vi "Start trigger export.vi"(4 "trig.pxi trig dst":i32, 6 "trig.export":T1, 7 "trig.dur":u32=25, 9 "delayed trigger":bool, 10 "synced trigger":bool, 11 "source trigger":bool) -> (0 "pxi3 ctr":u16, 1 "pxi1 ctr":u16, 2 "pxi0 ctr":u16, 3 "dst count":u16)   [LabVIEW 2019, in "FPGA Utility.lvlib"]
doc: "Handles trigger exporting to PXI tirg line"
uses:
  FPGA Utility.lvlib
  FPGA driver trigger destination.ctl
  <instrlib>/_niInstr/Basic Elements/v1/FPGA/Private/Count Up U16.vi
  <instrlib>/_niInstr/Basic Elements/v1/FPGA/niInstr Basic Elements v1 FPGA.lvlib
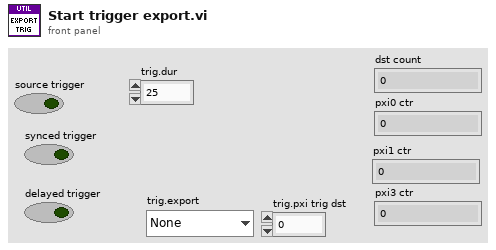
[diagram p1: front panel]
types:
  T1 = typedef "FPGA Utility.lvlib/FPGA driver trigger destination.ctl" = enum16{"None", "Source trig", "Synced trig", "Delayed sync"}
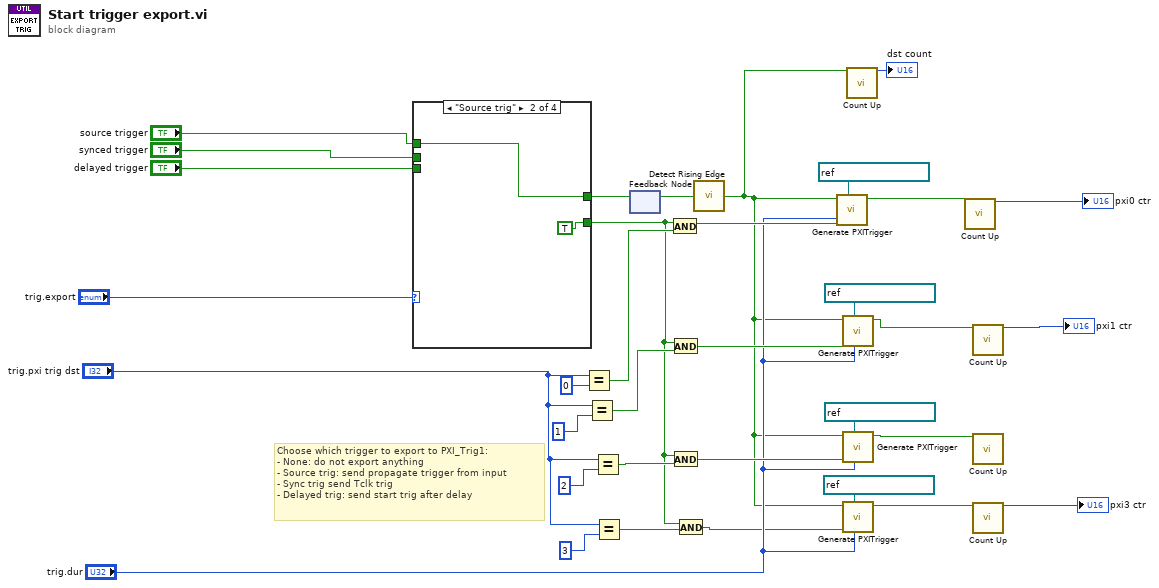
[diagram p0: block diagram]
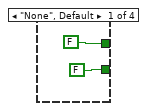
[diagram p2: hidden frame]
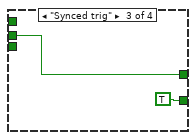
[diagram p3: hidden frame]
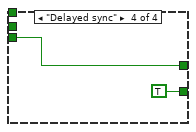
[diagram p4: hidden frame]
diagram:
  # "Choose which trigger to export to PXI_Trig1:\n- None: do not export anything\n- Source trig: send propagate trigger from input\n- Sync trig send Tclk trig\n- Delayed trig: send start trig after delay"
  n1 = case shown="\"Source trig\"" "trig.export" {
    tunnel: [FALSE TRUE TRUE TRUE] -> w6
    tunnel: [FALSE w38 w40 w41] -> w23
    tunnel: "source trigger" -> [_ w38 _ _]
    tunnel: "synced trigger" -> [_ _ w40 _]
    tunnel: "delayed trigger" -> [_ _ _ w41]
    frame "None", Default {
    }
    frame "Source trig" {
    }
    frame "Synced trig" {
    }
    frame "Delayed sync" {
    }
  }
  n2 = Equal?(x="trig.pxi trig dst", y=0) -> (x = y?=w31:bool)
  n3 = Equal?(x="trig.pxi trig dst", y=1) -> (x = y?=w33:bool)
  n4 = Equal?(x="trig.pxi trig dst", y=2) -> (x = y?=w7:bool)
  n5 = Equal?(x="trig.pxi trig dst", y=3) -> (x = y?=w5:bool)
  n6 = feedback #1() -> (w28:bool)  [unwired: 1 in]
  n7 = feedback-in #1(w23) -> ()
  n8 = And(x=w6, y=w31) -> (x .and. y?=w29:bool)
  n9 = And(x=w6, y=w33) -> (x .and. y?=w34:bool)
  n10 = And(x=w6, y=w7) -> (x .and. y?=w4:bool)
  n11 = And(x=w6, y=w5) -> (x .and. y?=w1:bool)
  n12 = call <instrlib>:"Detect Rising Edge.vi"("signal"=w28) -> ("edge detected"=w2:bool)  [unwired: 14 in]
  n13 = call "Generate PXITrigger.vi"("duration (ticks)"="trig.dur", "Trigger IO"=refnum<k21> "PXI_Trig0" ("FPGA I/O In"), "enable trigger generation"=w29, "send trigger"=w2) -> ("generated trig"=w19:bool)  [unwired: 7 in]
  n14 = call "Generate PXITrigger.vi"("duration (ticks)"="trig.dur", "Trigger IO"=refnum<k21> "PXI_Trig1" ("FPGA I/O In"), "enable trigger generation"=w34, "send trigger"=w2) -> ("generated trig"=w16:bool)  [unwired: 7 in]
  n15 = call "Generate PXITrigger.vi"("duration (ticks)"="trig.dur", "Trigger IO"=refnum<k21> "PXI_Trig2" ("FPGA I/O In"), "enable trigger generation"=w4, "send trigger"=w2) -> ("generated trig"=w15:bool)  [unwired: 7 in]
  n16 = call "Generate PXITrigger.vi"("duration (ticks)"="trig.dur", "Trigger IO"=refnum<k21> "PXI_Trig3" ("FPGA I/O In"), "enable trigger generation"=w1, "send trigger"=w2) -> ("generated trig"=w11:bool)  [unwired: 7 in]
  n17 = call-poly <instrlib>:"Count Up.vi"("increment"=w2) -> ("count out"=→"dst count":u16)  [unwired: 14 in]
  n18 = call-poly <instrlib>:"Count Up.vi"("increment"=w19) -> ("count out"=→"pxi0 ctr":u16)  [unwired: 14 in]
  n19 = call-poly <instrlib>:"Count Up.vi"("increment"=w16) -> ("count out"=→"pxi1 ctr":u16)  [unwired: 14 in]
  n20 = call-poly <instrlib>:"Count Up.vi"("increment"=w15) -> ()  [unwired: 14 in, 1 out]
  n21 = call-poly <instrlib>:"Count Up.vi"("increment"=w11) -> ("count out"=→"pxi3 ctr":u16)  [unwired: 14 in]
